vi "Shoot.vi"(2 "Shoot":bool=TRUE) -> ()   [LabVIEW 2016]
uses:
  <vilib>/Rock Robotics/WPI/SafetyOutput/WPI_SafetyOutputConfigMenu.ctl
  Global 2.vi
  <vilib>/gmath/NI_Gmath.lvlib
panel:
  in  "Adjustment X":dbl[](array[numeric])=[-3400.0, -3100.0, -2750.0, -2430.0, -2080.0, -1710.0, -1330.0, -950.0, -580.0, -210.0, 0.0, 210.0, 580.0, 950.0, 1330.0, 1710.0, 2080.0, 2430.0, 2750.0, 3100.0, 3400.0]
  in  "Adjustment Y":dbl[](array[numeric])=[-1.0, -0.9, -0.8, -0.7, -0.6, -0.5, -0.4, -0.3, -0.2, -0.1, 0.0, 0.1, 0.2, 0.3, 0.4, 0.5, 0.6, 0.7, 0.8, 0.9, 1.0] format="%_6g"
  out "Waveform Chart":cluster{dbl}(graph)={2565.46875}
  out "Motor Effort":dbl=0.17108041660508766
  out "Adjustment":dbl=-0.27365642550017555
  out "RPM":dbl=2565.46875
  in  "kP":dbl=0.8 format="%#_13g"
  in  "kD":dbl=0.06 format="%#_13g"
  in  "Y":dbl[](array[numeric])=[0.0, 0.1, 0.2, 0.3, 0.4, 0.5, 0.6, 0.7, 0.8, 0.9, 1.0] format="%_6g"
  in  "X":dbl[](array[numeric])=[0.0, 210.0, 580.0, 950.0, 1330.0, 1710.0, 2080.0, 2430.0, 2750.0, 3100.0, 3400.0]
  in  "RPM Target BB":dbl=1500.0
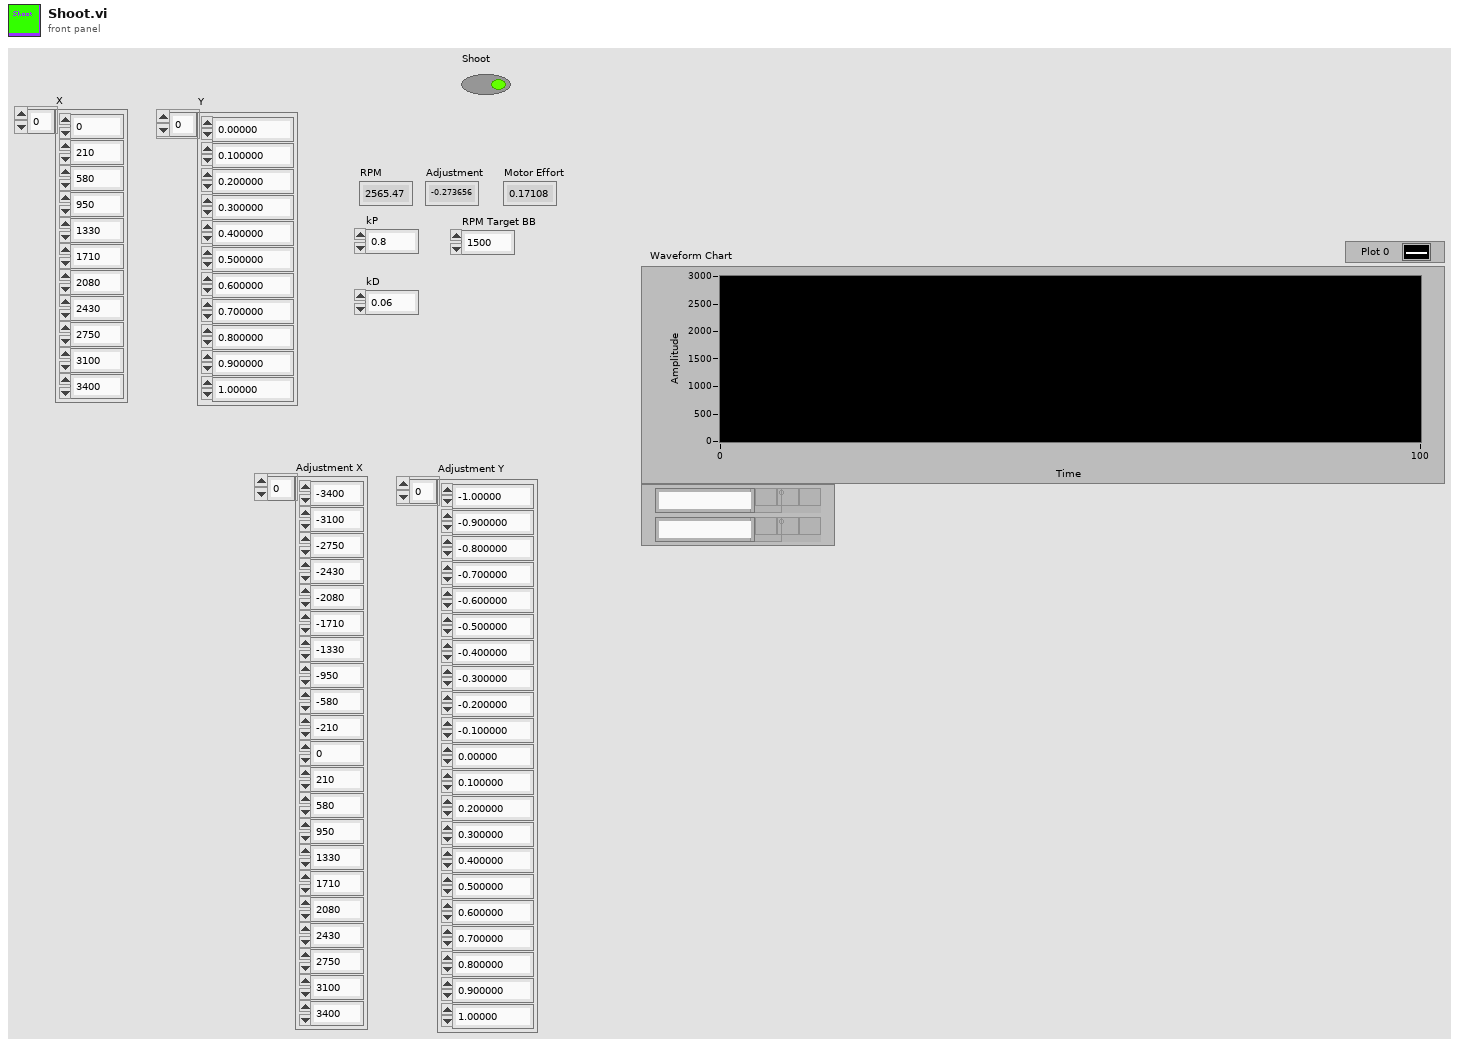
[diagram p1: front panel]
types:
  T1 = typedef "WPI_SafetyOutputConfigMenu.ctl" = enum16{"Enable", "Disable"}
  T2 = typedef "WPI_MotorControlDeviceRef.ctl" = cluster{"DeviceStatus":errorcluster, "Type":T3, "PWM":cluster{"PWM Channel":T4, "DeadBand":T5}, "CAN":cluster{"Device Number":u8, "SetOutput VI Ref":variant, "GetOutput VI Ref":variant, "Enable VI Ref":variant, "Disable VI Ref":variant, "Data":variant}, "Invert":bool}
  T3 = typedef "WPI_MotorControlType.ctl" = enum16{"PWM", "CAN"}
  T4 = typedef "FPGA_DIOPWMChannel.ctl" = enum8{"PWM 0", "PWM 1", "PWM 2", "PWM 3", "PWM 4", "PWM 5", "PWM 6", "PWM 7", "PWM 8", "PWM 9", "PWM MXP 0", "PWM MXP 1", "PWM MXP 2", "PWM MXP 3", "PWM MXP 4", "PWM MXP 5", "PWM MXP 6", "PWM MXP 7", "PWM MXP 8", "PWM MXP 9", "Invalid"}
  T5 = typedef "WPI_PWMDeadband.ctl" = cluster{"Name":string, "maxPositivePwm":i32, "minPositivePwm":i32, "centerPwm":i32, "maxNegativePwm":i32, "minNegativePwm":i32, "angularRange":u16}
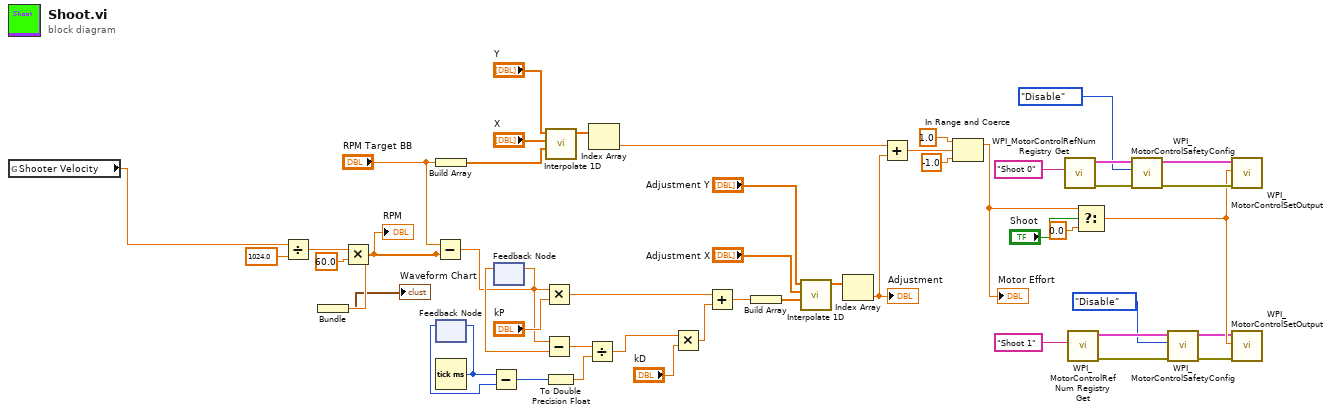
[diagram p0: block diagram]
diagram:
  n1 = global read "Global 2.vi" "Shooter Velocity"() -> (w12:dbl)
  n2 = Divide(x=w12, y=1024.0) -> (x/y=w47:dbl)
  n3 = Multiply(x=w47, y=60.0) -> (x*y=w18:dbl)
  "RPM" <- w18
  n4 = Bundle(w18) -> (→"Waveform Chart":cluster{dbl})  [unwired: 1 in]
  n5 = Subtract(x="RPM Target BB", y=w18) -> (x-y=w20:dbl)
  n6 = Build Array("RPM Target BB") -> (w45:dbl[])
  n7 = feedback #1() -> (w41:u32)  [unwired: 1 in]
  n8 = Tick Count (ms)() -> (millisecond timer value=w42:u32)
  n9 = feedback-in #1(w42) -> ()
  n10 = Subtract(x=w42, y=w41) -> (x-y=w39:u32)
  n11 = feedback #2() -> (w43:dbl)  [unwired: 1 in]
  n12 = feedback-in #2(w20) -> ()
  n13 = Multiply(x=w20, y="kP") -> (x*y=w33:dbl)
  n14 = Subtract(x=w20, y=w43) -> (x-y=w40:dbl)
  n15 = call <vilib>:"Interpolate 1D.vi"("xi"=w45, "X"="X", "Y"="Y") -> ("yi"=w44:dbl[])  [unwired: 6 in, 2 out]
  n16 = To Double Precision Float(number=w39) -> (double precision float=w38:dbl)
  n17 = Divide(x=w40, y=w38) -> (x/y=w37:dbl)
  n18 = Index Array(array=w44) -> (element=w31:dbl)  [unwired: 1 in]
  n19 = Multiply(x=w37, y="kD") -> (x*y=w32:dbl)
  n20 = Add(x=w33, y=w32) -> (x+y=w26:dbl)
  n21 = Build Array(w26) -> (w29:dbl[])
  n22 = call <vilib>:"Interpolate 1D.vi"("xi"=w29, "X"="Adjustment X", "Y"="Adjustment Y") -> ("yi"=w30:dbl[])  [unwired: 6 in, 2 out]
  n23 = Index Array(array=w30) -> (element=w25:dbl)  [unwired: 1 in]
  "Adjustment" <- w25
  n24 = Add(x=w31, y=w25) -> (x+y=w24:dbl)
  n25 = In Range and Coerce(upper limit=1.0, x=w24, lower limit=-1.0 ("upper limit")) -> (coerced(x)=w21:dbl)  [unwired: 1 out]
  "Motor Effort" <- w21
  n26 = call <vilib>:"WPI_MotorControlRefNum Registry Get.vi"("refnum name"="Shoot 0") -> ("error out"=w1:errorcluster, "MotorControlDevRef"=w11:T2)  [unwired: 9 in]
  n27 = call <vilib>:"WPI_MotorControlRefNum Registry Get.vi"("refnum name"="Shoot 1") -> ("error out"=w6:errorcluster, "MotorControlDevRef"=w7:T2)  [unwired: 9 in]
  n28 = Select(t=w21, s="Shoot", f=0.0) -> (s? t:f=w5:dbl)
  n29 = call <vilib>:"WPI_MotorControlSafetyConfig.vi"("error in (no error)"=w1, "mode"=WPI_SafetyOutputConfigMenu."Disable", "MotorControlDevRef"=w11) -> ("error out"=w9:errorcluster, "MotorControlDevRef"=w10:T2)  [unwired: 7 in]
  n30 = call <vilib>:"WPI_MotorControlSafetyConfig.vi"("error in (no error)"=w6, "mode"=WPI_SafetyOutputConfigMenu."Disable", "MotorControlDevRef"=w7) -> ("error out"=w3:errorcluster, "MotorControlDevRef"=w4:T2)  [unwired: 7 in]
  n31 = call <vilib>:"WPI_MotorControlSetOutput.vi"("error in (no error)"=w9, "Output"=w5, "MotorControlDevRef"=w10) -> ()  [unwired: 6 in, 3 out]
  n32 = call <vilib>:"WPI_MotorControlSetOutput.vi"("error in (no error)"=w3, "Output"=w5, "MotorControlDevRef"=w4) -> ()  [unwired: 6 in, 3 out]
